vi "WeightSensor.vi"() -> ()   [LabVIEW 2022 SP3]
uses:
  <vilib>/DAQmx/read.llb/DAQmx Read (Analog DBL 1Chan 1Samp).vi
  <vilib>/DAQmx/create/channels.llb/DAQmx Create Channel (AI-Voltage-Basic).vi
  <vilib>/DAQmx/miscellaneous.llb/DAQmx Fill In Error Info.vi
panel:
  out "Weight Range":dbl(knob) scale=0.0..1500.0
  in  "physical channels":tag
  out "Meter":dbl(knob) scale=4.0..10.0
  in  "stop":bool
  # "Range (g)"
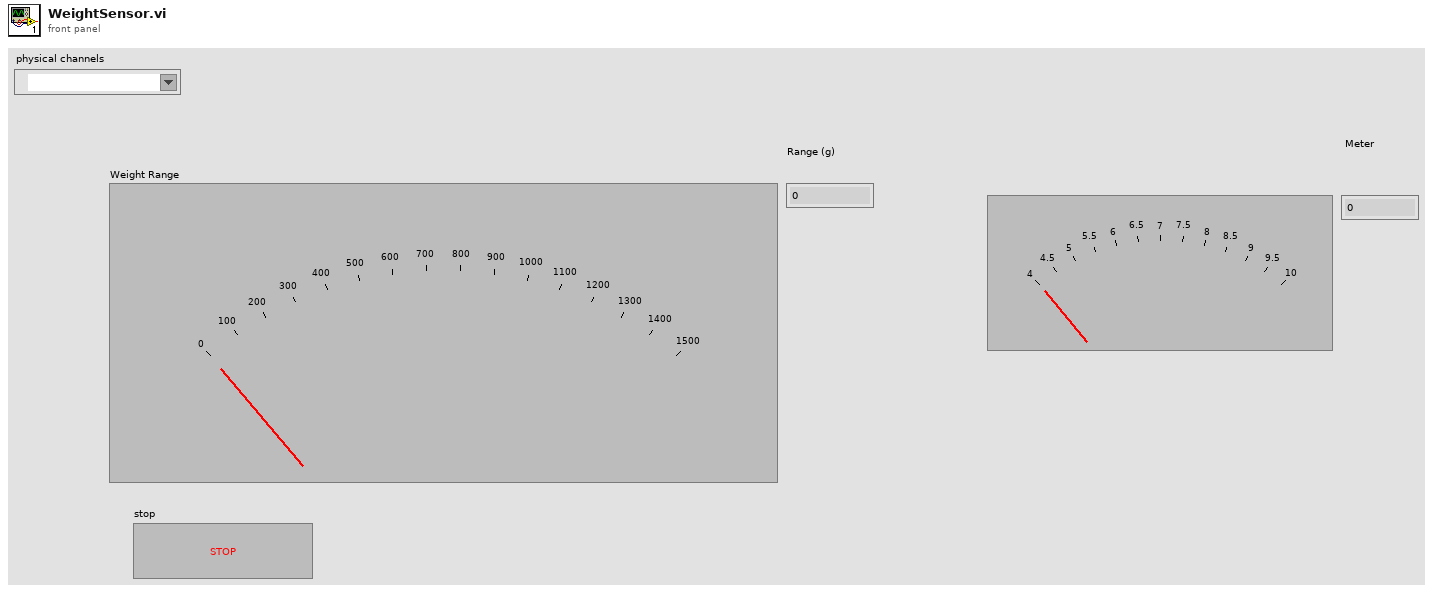
[diagram p1: front panel]
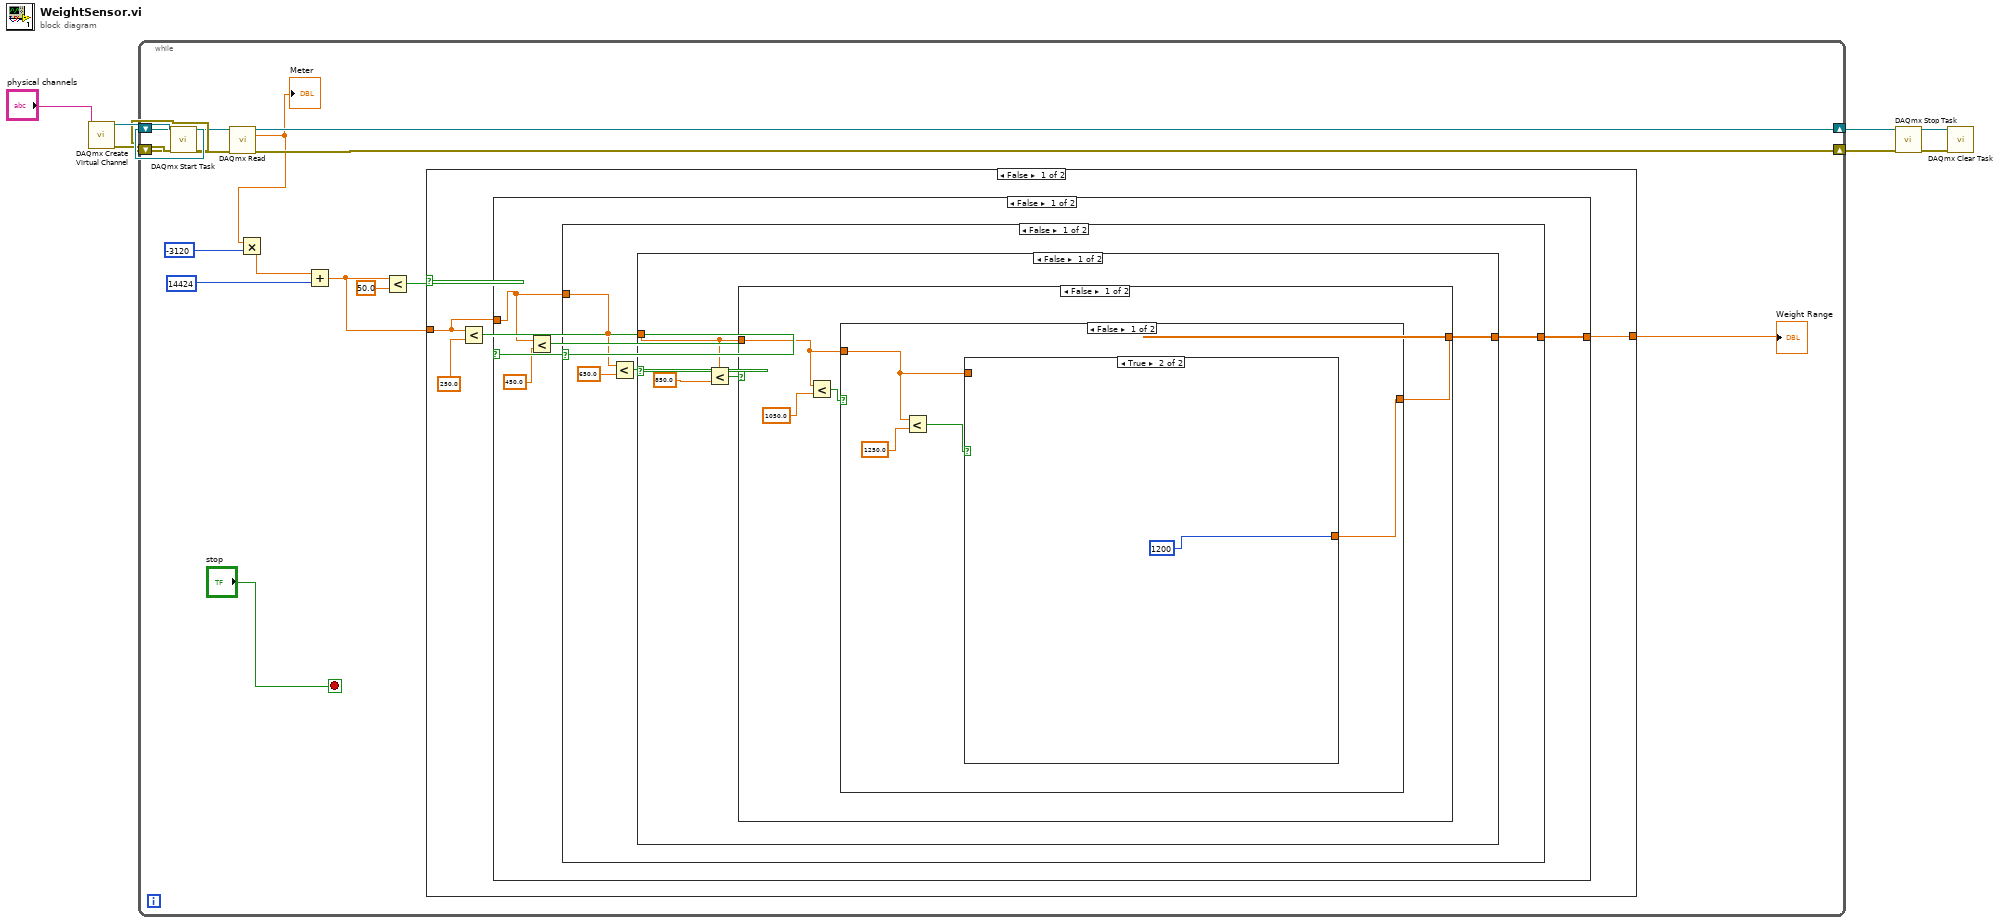
[diagram p0: block diagram]
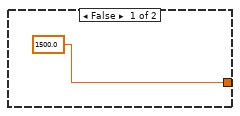
[diagram p2: hidden frame]
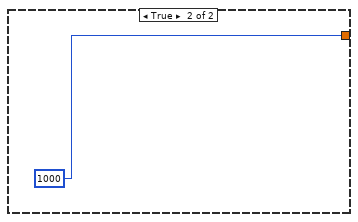
[diagram p3: hidden frame]
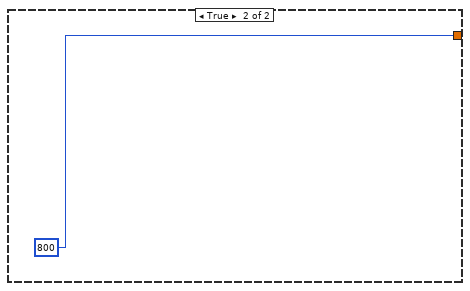
[diagram p4: hidden frame]
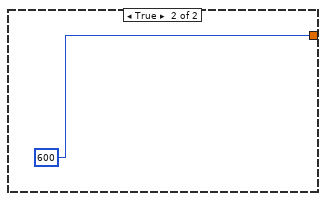
[diagram p5: hidden frame]
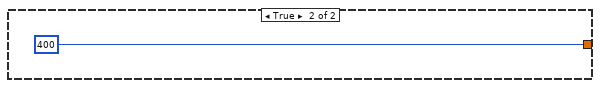
[diagram p6: hidden frame]
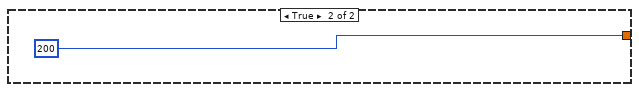
[diagram p7: hidden frame]
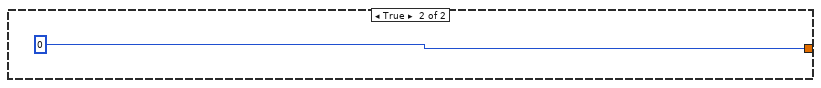
[diagram p8: hidden frame]
diagram:
  n1 = call-poly <vilib>:"DAQmx Create Virtual Channel.vi"("physical channels"="physical channels") -> ("task out"=w9:refnum<k21>, "error out"=w5:errorcluster)  [unwired: 13 in]
  n2 = call <vilib>:"DAQmx Start Task.vi"("task/channels in"=w9, "error in"=w5) -> ("task out"=w8:refnum<k21>, "error out"=w4:errorcluster)  [unwired: 12 in]
  n3 = while {
    shift-right: [w21] -> w7
    shift-left: w8 -> [w22]
    shift-right: [w19] -> w3
    shift-left: w4 -> [w20]
    stop <- "stop" stop-if-true
    n4 = call-poly <vilib>:"DAQmx Read.vi"("task/channels in"=w22, "error in"=w20) -> ("task out"=w21:refnum<k21>, "data"=w16:dbl, "error out"=w19:errorcluster)  [unwired: 11 in]
    "Meter" <- w16
    n5 = Multiply(x=w16, y=-3120) -> (x*y=w15:dbl)
    n6 = Add(x=w15, y=14424) -> (x+y=w10:dbl)
    n7 = Less?(x=w10, y=50.0) -> (x < y?=w12:bool)
    n8 = case shown="False" w12 {
      tunnel: [w24 0] -> w11
      tunnel: w10 -> [w23 _]
      frame False {
        n9 = Less?(x=w23, y=250.0) -> (x < y?=w25:bool)
        n10 = case shown="False" w25 {
          tunnel: [w29 200] -> w24
          tunnel: w23 -> [w27 _]
          frame False {
            n11 = Less?(x=w27, y=450.0) -> (x < y?=w28:bool)
            n12 = case shown="False" w28 {
              tunnel: [w31 400] -> w29
              tunnel: w27 -> [w32 _]
              frame False {
                n13 = Less?(x=w32, y=650.0) -> (x < y?=w33:bool)
                n14 = case shown="False" w33 {
                  tunnel: w32 -> [w36 _]
                  tunnel: [w35 600] -> w31
                  frame False {
                    n15 = Less?(x=w36, y=850.0) -> (x < y?=w37:bool)
                    n16 = case shown="False" w37 {
                      tunnel: w36 -> [w40 _]
                      tunnel: [w39 800] -> w35
                      frame False {
                        n17 = Less?(x=w40, y=1050.0) -> (x < y?=w41:bool)
                        n18 = case shown="False" w41 {
                          tunnel: [w43 1000] -> w39
                          tunnel: w40 -> [w44 _]
                          frame False {
                            n19 = Less?(x=w44, y=1250.0) -> (x < y?=w45:bool)
                            n20 = case shown="True" w45 {
                              tunnel: [1500.0 ("y") 1200] -> w43
                              tunnel: w44 -> [_ _]
                              frame False {
                              }
                              frame True {
                              }
                            }
                          }
                          frame True {
                          }
                        }
                      }
                      frame True {
                      }
                    }
                  }
                  frame True {
                  }
                }
              }
              frame True {
              }
            }
          }
          frame True {
          }
        }
      }
      frame True {
      }
    }
    "Weight Range" <- w11
  }
  n21 = call <vilib>:"DAQmx Stop Task.vi"("task/channels in"=w7, "error in"=w3) -> ("task out"=w6:refnum<k21>, "error out"=w2:errorcluster)  [unwired: 12 in]
  n22 = call <vilib>:"DAQmx Clear Task.vi"("task in"=w6, "error in"=w2) -> ()  [unwired: 13 in, 1 out]
